vi "sequencerGlobVars.vi"() -> ()   [LabVIEW 2014]
uses:
  sequencerState.ctl
panel:
  out "currentScan":i32=-1
  out "currentStep":i32=-1
  in  "pause":bool
  in  "hostConfirmsHzOffsetIsSet":bool
  in  "cmdByHost":T1
  out "seqState":T1
  in  "halt":bool
  in  "abort":bool
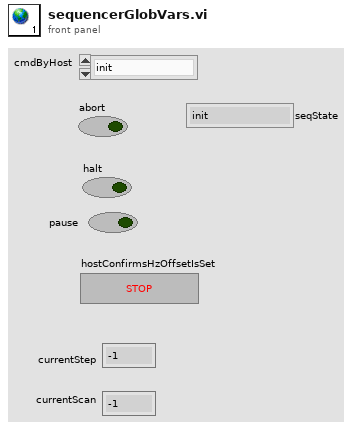
[diagram p1: front panel]
types:
  T1 = typedef "sequencerState.ctl" = enum16{"init", "idle", "measureOffset", "measureTrack", "measComplete", "error"}
diagram:
